vi "build_commands_2017.11.14.vi"(11 "T1_parameters":T1) -> (3 "instructions_array":T2(array[cluster]))   [LabVIEW 2014]
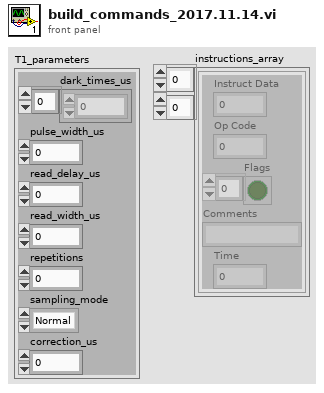
[diagram p1: front panel]
types:
  T1 = cluster{"dark_times_us":dbl[], "pulse_width_us":dbl, "read_delay_us":dbl, "read_width_us":dbl, "repetitions":i32, "sampling_mode":enum16{"Normal", "Sweep"}, "correction_us":dbl}
  T2 = cluster{"Instruct Data":i32, "Op Code":i32, "Flags":bool[], "Comments":string, "Time":dbl}[][]
  T3 = cluster{"Instruct Data":i32, "Op Code":i32, "Flags":bool[], "Comments":string, "Time":dbl}[]
  T4 = cluster{"Instruct Data":i32, "Op Code":i32, "Flags":bool[], "Comments":string, "Time":dbl}
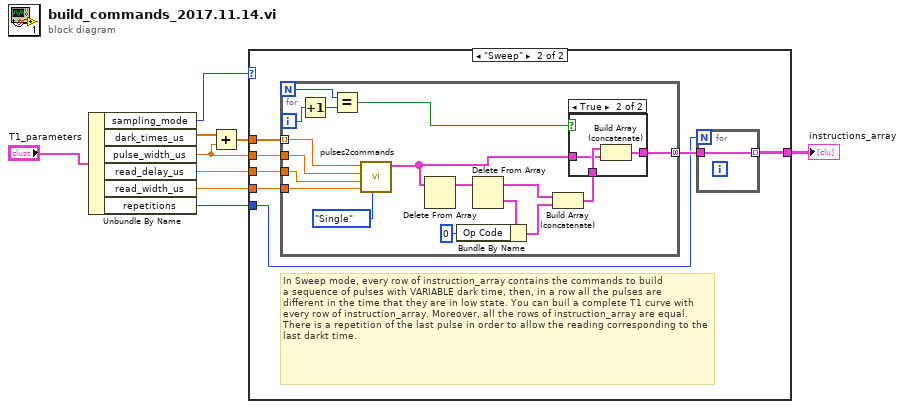
[diagram p0: block diagram]
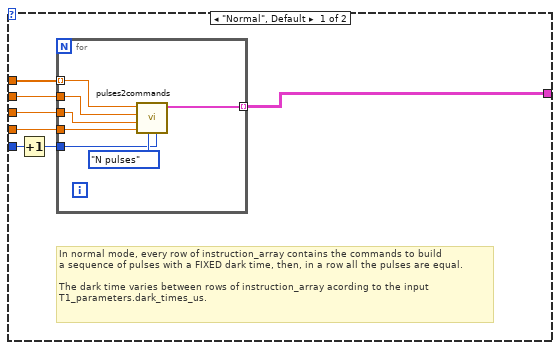
[diagram p2: hidden frame]
diagram:
  n1 = Unbundle By Name("T1_parameters") -> ("sampling_mode"=w2:enum16{"Normal", "Sweep"}, "dark_times_us"=w4:dbl[], "pulse_width_us"=w6:dbl, "read_delay_us"=w7:dbl, "read_width_us"=w8:dbl, "repetitions"=w9:i32)
  n2 = Add(x=w4, y=w6) -> (x+y=w5:dbl[])
  n3 = case shown="\"Sweep\"" w2 {
    tunnel: w5 -> [w12 w30]
    tunnel: w6 -> [w13 w29]
    tunnel: w7 -> [w14 w28]
    tunnel: w8 -> [w15 w27]
    tunnel: w9 -> [w16 w25]
    tunnel: [w10 w24] -> w3
    frame "Normal", Default {
      # "In normal mode, every row of instruction_array contains the commands to build \na sequence of pulses with a FIXED dark time, then, in a row all the pulses are equal.\n\nThe dark time varies between rows of instruction_array acording to the input\nT1_parameters.dark_times_us."
      n4 = Increment(x=w16) -> (x+1=w11:i32)
      n5 = for {
        tunnel: w11 -> [w22]
        tunnel: w15 -> [w21]
        tunnel: w14 -> [w20]
        tunnel: w13 -> [w19]
        tunnel: w12 -> [w18] mode=indexing
        tunnel: [w17] -> w10 mode=indexing
        n6 = call "pulses2commands.vi"("N_pulses"=w22, "running_mode"=enum16{"Continuous", "Single", "N pulses"}."N pulses", "read_width_us"=w21, "read_delay_us"=w20, "pulse_width_us"=w19, "pulse_period_us"=w18) -> ("instructions_array"=w17:T3)  [unwired: 4 in, 1 out]
      }
    }
    frame "Sweep" {
      # "In Sweep mode, every row of instruction_array contains the commands to build \na sequence of pulses with VARIABLE dark time, then, in a row all the pulses are \ndifferent in the time that they are in low state. You can buil a complete T1 curve with every row of instruction_array. Moreover, all the rows of instruction_array are equal.\nThere is a repetition of the last pulse in order to allow the reading corresponding to the last darkt time."
      n7 = for {
        N -> [w41]
        tunnel: w30 -> [w48] mode=indexing
        tunnel: w29 -> [w47]
        tunnel: w28 -> [w46]
        tunnel: w27 -> [w45]
        tunnel: [w32] -> w26 mode=concatenating
        i -> [w43]
        n8 = Increment(x=w43) -> (x+1=w42:i32)
        n9 = Equal?(x=w41, y=w42) -> (x = y?=w35:bool)
        n10 = call "pulses2commands.vi"("running_mode"=enum16{"Continuous", "Single", "N pulses"}."Single", "read_width_us"=w45, "read_delay_us"=w46, "pulse_width_us"=w47, "pulse_period_us"=w48) -> ("instructions_array"=w33:T3)  [unwired: 5 in, 1 out]
        n11 = Delete From Array(array=w33) -> (array with subset deleted=w38:T3)  [unwired: 2 in, 1 out]
        n12 = Delete From Array(array=w38) -> (deleted portion=w37:T4, array with subset deleted=w36:T3)  [unwired: 2 in]
        n13 = Bundle By Name(cluster=w37, "Op Code"=0) -> (w39:T4)
        n14 = Build Array (concatenate)(w36, w39) -> (w34:T3)
        n15 = case shown="True" w35 {
          tunnel: w34 -> [w49 w52]
          tunnel: [w49 w51] -> w32
          tunnel: w33 -> [_ w50]
          frame False {
          }
          frame True {
            n16 = Build Array (concatenate)(w52, w50) -> (w51:T3)
          }
        }
      }
      n17 = for {
        N: w25 -> [_]
        tunnel: w26 -> [w31]
        tunnel: [w31] -> w24 mode=indexing
      }
    }
  }
  "instructions_array" <- w3
